vi "Write TS Front Panel Refnum.vi"(8 "error in (no error)":errorcluster, 10 "TS Front Panel Refnum":refnum<vi>, 11 "UI Display TS Panel in":refnum<class "UI Display TS Panel.lvclass">) -> (0 "error out":errorcluster, 3 "UI Display TS Panel out":refnum<class "UI Display TS Panel.lvclass">)   [LabVIEW 2019, in "User Interface Process.lvlib" / "UI Display TS Panel.lvclass"]
uses:
  UI Display TS Panel.lvclass
  UI Display TS Panel.lvclass/UI Display TS Panel.ctl
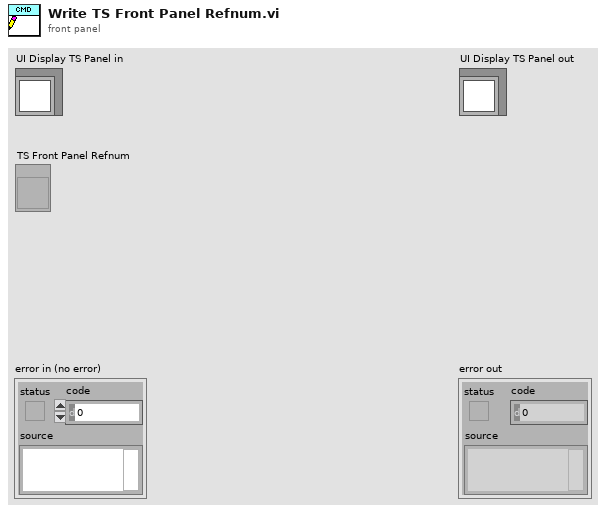
[diagram p1: front panel]
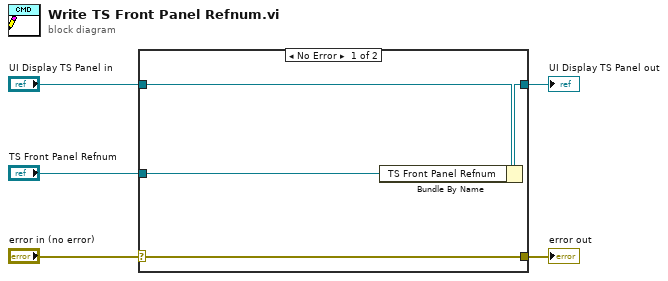
[diagram p0: block diagram]
diagram:
  n1 = case shown="No Error" "error in (no error)" {
    selector: "error in (no error)" -> [w9 w10]
    tunnel: [w9 w10] -> w4
    tunnel: [w7 w11] -> w2
    tunnel: "UI Display TS Panel in" -> [w8 w11]
    tunnel: "TS Front Panel Refnum" -> [w6 _]
    frame No Error {
      n2 = Bundle By Name(cluster=w8, "TS Front Panel Refnum"=w6) -> (w7:refnum<class "UI Display TS Panel.lvclass">)
    }
    frame Error {
    }
  }
  "error out" <- w4
  "UI Display TS Panel out" <- w2
